vi "Set ReadRate.vi"(10 "ReadRate":dbl format="%#_g Hz", 11 "Worker in":refnum<class "Camera Worker.lvclass">) -> (3 "Worker out":refnum<class "Camera Worker.lvclass">)   [LabVIEW 2025, in "Camera Worker.lvlib" / "Camera Worker.lvclass"]
uses:
  Camera Worker.lvclass
  Camera Worker.lvclass/Camera Worker.ctl
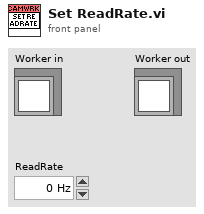
[diagram p1: front panel]
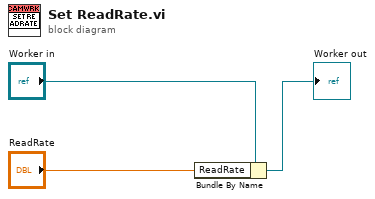
[diagram p0: block diagram]
diagram:
  n1 = Bundle By Name(cluster="Worker in", "ReadRate"="ReadRate") -> (→"Worker out":refnum<class "Camera Worker.lvclass">)
